vi "ASI_Disable_Enable_Controls.vi"(2 "Enable Z":bool, 3 "error in":errorcluster, 4 "Enable XY":bool, 5 "VISA resource name":refnum<visa-resource-name>) -> (0 "error out":errorcluster, 1 "VISA resource name out":refnum<visa-resource-name>)   [LabVIEW 2018]
panel:
  out "Serial Settings:Number of Bytes at Serial Port":u32
  out "read buffer":string
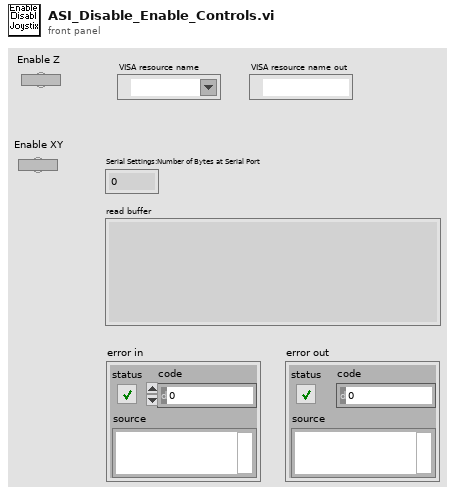
[diagram p1: front panel]
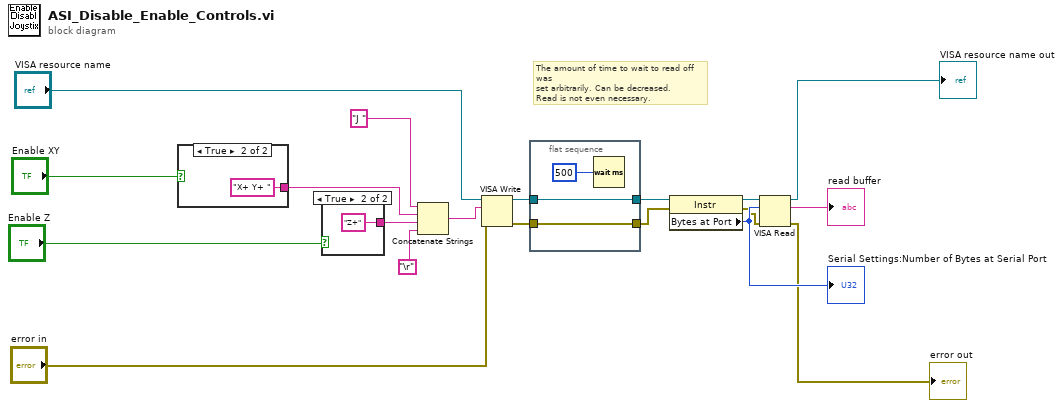
[diagram p0: block diagram]
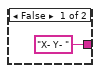
[diagram p2: hidden frame]
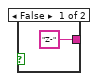
[diagram p3: hidden frame]
diagram:
  # "The amount of time to wait to read off was \nset arbitrarily. Can be decreased.  \nRead is not even necessary."
  n1 = case shown="True" "Enable XY" {
    tunnel: ["X- Y- " "X+ Y+ "] -> w1
    frame False {
    }
    frame True {
    }
  }
  n2 = case shown="True" "Enable Z" {
    tunnel: ["Z-" "Z+"] -> w19
    frame False {
    }
    frame True {
    }
  }
  n3 = Concatenate Strings("J " ("string"), w1, w19, "\r") -> (w18:string)
  n4 = VISA Write(VISA resource name="VISA resource name", write buffer=w18, error in (no error)="error in") -> (VISA resource name out=w13:refnum<visa-resource-name>, error out=w7:errorcluster)  [unwired: 1 out]
  n5 = flat-sequence {
    tunnel: [w26] -> w14
    tunnel: w13 -> [w26]
    tunnel: [w24] -> w8
    tunnel: w7 -> [w24]
    frame #0 {
      n6 = Wait (ms)(milliseconds to wait=u32 500) -> ()  [unwired: 1 out]
    }
  }
  n7 = property class="Instr"(reference=w14, error in=w8) -> (reference out=w17:refnum<visa-resource-name>, error out=w6:errorcluster, "Bytes at Port"=w16:u32)
  "Serial Settings:Number of Bytes at Serial Port" <- w16
  n8 = VISA Read(VISA resource name=w17, byte count=w16, error in (no error)=w6) -> (VISA resource name out=→"VISA resource name out":refnum<visa-resource-name>, read buffer=→"read buffer":string, error out=→"error out":errorcluster)  [unwired: 1 out]
